vi "PH_Beckhoff_StepMot.Action Configure.vi"(0 "VI in":refnum<vi>, 5 "error in":errorcluster) -> (14 "VI out":refnum<vi>, 19 "error out":errorcluster)   [LabVIEW 2014, in "PH_Beckhoff_StepMot.lvlib"]
uses:
  PH_Beckhoff_StepMot.lvlib
  PH_Beckhoff/PH_Beckhoff.lvlib
  PH_Basics/PH_Stepmotor_BaseClass/PH_Stepmotor_BaseClass.lvlib
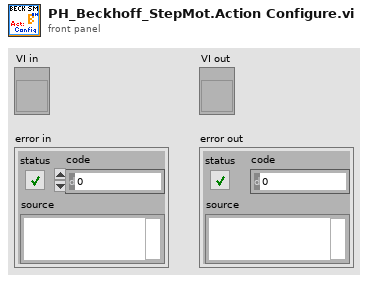
[diagram p1: front panel]
types:
  T1 = typedef "PH_Beckhoff.lvlib/PH_Beckhoff.i attribute.ctl" = cluster{"GUI Refs":T2, "operation?":bool, "Default Prdc Interval":i32, "Connection":T3, "AMS Net ID":T4, "Klemmencluster: # of":T5, "Values":T6, "IP":string, "Description":string, "configured?":bool, "Change Manager":cluster{"Detemination wanted?":bool, "Values changed at":cluster{"Sonderklemmen Inputs":i32[], "Analog Inputs":i32[], "Analog Outputs":i32[], "Digital Inputs":i32[], "Digital Outputs":i32[]}}, "Difference to handle an analog input as change":u32}
  T2 = typedef "PH_Beckhoff.lvlib/PH_Beckhoff.GUI Refs.ctl" = cluster{"ADS Error":refnum<vi>, "Values":refnum<vi>, "configured?":refnum<vi>, "Connection":refnum<vi>, "IP":refnum<vi>, "Prdc Int [ms]":refnum<vi>}
  T3 = typedef "PH_Beckhoff.lvlib/PH_Beckhoff.Connectivity.ctl" = cluster{"DLL?":bool, "Port?":bool, "Client?":bool, "Ping?":bool, "unsuccessful Pings":u32}
  T4 = typedef "Beckhoff - Driver np.lvlib/Beckhoff Access.ctl" = cluster{"DLL path":path, "AMS Net ID":cluster{"1st # of IP":u8, "2nd # of IP":u8, "3rd # of IP":u8, "4th # of IP":u8, "In Port":u8, "Out Port":u8}}
  T5 = typedef "Beckhoff - Driver np.lvlib/Klemmendeclarer.ctl" = cluster{"Offset due to Sonderklemms":u32, "analog Inputs":u32, "analog Outputs":u32, "digital Input Bits":u32, "digital Output Bits":u32}
  T6 = typedef "PH_Beckhoff.lvlib/PH_Beckhoff.Values.ctl" = cluster{"Sonderklemmen Inputs":T7, "Analog Inputs":T8, "Analog Outputs":T10, "Digital Inputs":T11, "Digital Outputs":T12}
  T7 = typedef "PH_Beckhoff.lvlib/PH_Beckhoff.Sonderklemmen Inputs.ctl" = cluster{"Total Length":u32, "Name":string, "Value":u64, "Quality":bool, "Service ID":i32, "Offset":u32, "Length":u32}[]
  T8 = typedef "PH_Beckhoff.lvlib/PH_Beckhoff.Analog Inputs.ctl" = cluster{"Name":string, "Value":u32, "Quality":bool, "Service ID":i32, "Sca Type":T9}[]
  T9 = typedef "PH_Beckhoff.lvlib/PH_Beckhoff.Scaling Type.ctl" = enum16{"none", "0 ... 15 Bit -> 0 ... 5", "0 ... 15 Bit -> 0 ... 10", "0 ... 15 Bit -> 0 ... 25", "0 ... 15 Bit -> 4 ... 20", "0 ... 15 Bit -> 0 ... 1", "0 ... 15 Bit -> 0 ... 20000", "0 ... 15 Bit -> 0 ... 24000"}
  T10 = typedef "PH_Beckhoff.lvlib/PH_Beckhoff.Analog Outputs.ctl" = cluster{"Name":string, "Value":u32, "Quality":bool, "Wanted Value":u32, "Service ID":i32, "Sca Type":T9}[]
  T11 = typedef "PH_Beckhoff.lvlib/PH_Beckhoff.Digital Inputs.ctl" = cluster{"Name":string, "Value":bool, "Quality":bool, "Service ID":i32, "inverted?":bool}[]
  T12 = typedef "PH_Beckhoff.lvlib/PH_Beckhoff.Digital Outputs.ctl" = cluster{"Name":string, "Value":bool, "Quality":bool, "Wanted Value":bool, "Service ID":i32, "inverted?":bool}[]
  T13 = typedef "PH_Beckhoff_StepMot.lvlib/PH_Beckhoff_StepMot.i attribute.ctl" = cluster{"Axes Settings":T14[], "GUI Refs":cluster{"Axes Settings":refnum<vi>, "Stati":refnum<vi>}, "Get Beckhoff Settings":bool}
  T14 = typedef "PH_Beckhoff_StepMot.lvlib/PH_Beckhoff_StepMot.Axis Cluster.ctl" = cluster{"Step Motor Configuration":T15, "To set?":bool, "Endswitch inverted?":bool}
  T15 = typedef "Beckhoff - Driver np.lvlib/Beckhoff.Step Motor - Motor Configuration.ctl" = cluster{"Feature Register":T16, "I max A [mA]":dbl, "I max B [mA]":dbl, "v min":u32, "v max":u32, "a max":u32, "I hold [%]":u32, "Steps/qp":u32, "Feature Register 2":T17}
  T16 = typedef "Beckhoff - Driver np.lvlib/Beckhoff.Step Motor - Feature Register 1.ctl" = cluster{"en Auto Start":bool, "en Auto Stop":bool, "dis Wd Timer":bool, "OP Mode 1":bool, "OP Mode 2":bool, "Ramp Type":bool, "inv Pos Feedback":bool, "en User Cur Table":bool, "en Latch Evt Clr Pos":bool, "en Multi Latch Vals":bool, "en Sign Disp*":bool, "Feedback Type*":bool, "en neg Gate Lock*":bool, "en pos Gate Lock*":bool, "dis Enc Fltr*":bool, "en Counter Mode*":bool}
  T17 = typedef "Beckhoff - Driver np.lvlib/Beckhoff.Step Motor - Feature Register 2.ctl" = cluster{"rev Homing Dir":bool, "en Decac Ramp":bool, "Latch Reg Pos":bool, "Show Idle":bool, "dis Ref Input 1":bool, "dis Ref Input 2":bool, "en ext Auto Start":bool, "N/A":bool, "N/A":bool, "N/A":bool, "N/A":bool, "N/A":bool, "en Clr Proc Data":bool, "en Man Ecl Tolerce*":bool, "rev Dig Input 1":bool, "rev Dig Input 2":bool}
  T18 = typedef "PH_Stepmotor_BaseClass.lvlib/PH_Stepmotor_BaseClass.i attribute.ctl" = cluster{"Device Error":errorcluster, "Axes PSDB Thread":cluster{"Ref":refnum<vi>, "Q-Ref":refnum<queue>, "Data Status":T19}, "Axes":T20[], "Axes PSDB Infos":cluster{"GUI Name":string, "PSDB Instance ID":i32, "PSDB Status Service ID":i32, "Axis":i32, "Class":string}[], "GUI Refs":T25}
  T19 = typedef "PH_PSDBWriter.lvlib/PH_PSDBWriter.Data Status.ctl" = i16
  T20 = typedef "PH_Stepmotor_BaseClass.lvlib/PH_Stepmotor_BaseClass.Axis Attributes.ctl" = cluster{"Settings":T21, "Endswitch?":bool, "DIM Service IDs":T23, "Activity":T24, "Configured?":bool, "Position":cluster{"Current":i32, "Target":i32}, "Position to set":cluster{"New?":bool, "Wanted":i32}, "Stop?":bool, "Reset?":bool, "Move?":bool, "Nothing connected?":bool}
  T21 = typedef "PH_Stepmotor_BaseClass.lvlib/PH_Stepmotor_BaseClass.Axis Settings.ctl" = cluster{"Sign change":bool, "Width":dbl, "Calibration":dbl, "Unit":string, "Motor Type":T22, "Unit Width":string, "Unit CF":string}
  T22 = typedef "PH_Stepmotor_BaseClass.lvlib/PH_Stepmotor_BaseClass.Motor Type.ctl" = enum16{"Unspecific", "OWIS 49.120.2633", "OWIS 49.060.1033", "OWIS 43.040.2558", "Diamond Motion 2200 series", "OWIS 49.120.266B.MV6", "Calorimeter", "Linear Stage 1", "MICOS VT-80", "MICOS VT-80 S", "Standa Rotstage nt0.95A", "PUF RA 320.200", "PUF RA 800.200", "PUF RA 800.400", "PUF RA 400.50", "1324.nn.800.50", "1324.n9c.800.50", "1324.nn.320.200", "1324.nn.400.200", "1324.nn.800.200", "1324.nn.400.50", "1324.8c9c.800.50", "1324.8c9c.400.200"}
  T23 = typedef "PH_Stepmotor_BaseClass.lvlib/PH_Stepmotor_BaseClass.Axis DIM Service IDs.ctl" = cluster{"Settings":i32, "Information":i32}
  T24 = typedef "PH_Stepmotor_BaseClass.lvlib/PH_Stepmotor_BaseClass.Axis Activity.ctl" = enum16{"No Information", "stopped", "running", "Failure", "Alarm", "stopped at backward ES", "stopped at foreward ES"}
  T25 = typedef "PH_Stepmotor_BaseClass.lvlib/PH_Stepmotor_BaseClass.GUI Refs.ctl" = cluster{"Axes Configuration":refnum<vi>, "Device Error":refnum<vi>, "Axes PSDB Infos":refnum<vi>}
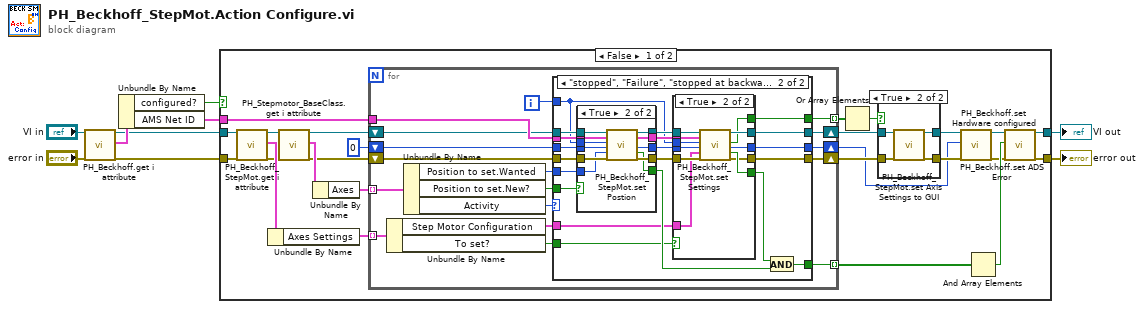
[diagram p0: block diagram]
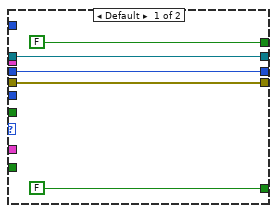
[diagram p3: hidden frame]
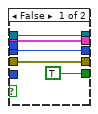
[diagram p4: hidden frame]
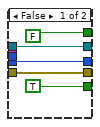
[diagram p5: hidden frame]
diagram:
  n1 = call "PH_Beckhoff.get i attribute.vi"("i ref in"="VI in", "error in (no error)"="error in") -> ("i ref out"=w4:refnum<vi>, "i attribute"=w7:T1, "error out"=w2:errorcluster)  [unwired: 15 in]
  n2 = Unbundle By Name(w7) -> ("configured?"=w1:bool, "AMS Net ID"=w6:T4)
  n3 = case shown="False" w1 {
    tunnel: [w31 w115] -> w9
    tunnel: [w30 w116] -> w8
    tunnel: w6 -> [w27 _]
    tunnel: w4 -> [w16 w116]
    tunnel: w2 -> [w13 w115]
    frame False {
      n4 = call "PH_Beckhoff_StepMot.get i attribute.vi"("i ref in"=w16, "error in (no error)"=w13) -> ("i ref out"=w15:refnum<vi>, "i attribute"=w32:T13, "error out"=w12:errorcluster)  [unwired: 15 in]
      n5 = Unbundle By Name(w32) -> ("Axes Settings"=w33:T14[])
      n6 = call "PH_Stepmotor_BaseClass.get i attribute.vi"("i ref in"=w15, "error in (no error)"=w12) -> ("i ref out"=w14:refnum<vi>, "i attribute"=w18:T18, "error out"=w11:errorcluster)  [unwired: 15 in]
      n7 = Unbundle By Name(w18) -> ("Axes"=w17:T20[])
      n8 = for {
        tunnel: w27 -> [w57]
        shift-right: [w53] -> w25
        shift-left: w11 -> [w56]
        shift-right: [w54] -> w10
        shift-left: 0 ("ADS Error out") -> [w55]
        tunnel: w33 -> [w43] mode=indexing
        shift-right: [w51] -> w22
        shift-left: w14 -> [w52]
        tunnel: [w44] -> w34 mode=indexing
        tunnel: [w50] -> w20 mode=indexing
        tunnel: w17 -> [w49] mode=indexing
        i -> [w46]
        n9 = Unbundle By Name(w43) -> ("Step Motor Configuration"=w42:T15, "To set?"=w41:bool)
        n10 = Unbundle By Name(w49) -> ("Position to set.Wanted"=w48:i32, "Position to set.New?"=w47:bool, "Activity"=w45:T24)
        n11 = case shown="\"stopped\", \"Failure\", \"stopped at backward ES\", \"stopped at foreward ES\"" w45 {
          tunnel: w57 -> [_ w78]
          tunnel: w56 -> [w61 w73]
          tunnel: w55 -> [w59 w77]
          tunnel: [w59 w82] -> w54
          tunnel: w42 -> [_ w64]
          tunnel: [w61 w81] -> w53
          tunnel: w52 -> [w62 w72]
          tunnel: [w62 w80] -> w51
          tunnel: [FALSE w66] -> w44
          tunnel: w46 -> [_ w68]
          tunnel: [FALSE ("Settings changed?") w79] -> w50
          tunnel: w48 -> [_ w76]
          tunnel: w47 -> [_ w69]
          tunnel: w41 -> [_ w63]
          frame Default {
          }
          frame "stopped", "Failure", "stopped at backward ES", "stopped at foreward ES" {
            n12 = case shown="True" w69 {
              tunnel: w78 -> [w85 w93]
              tunnel: w77 -> [w84 w92]
              tunnel: w68 -> [_ w94]
              tunnel: w76 -> [_ w91]
              tunnel: [w87 w97] -> w75
              tunnel: [w86 w95] -> w74
              tunnel: w73 -> [w86 w96]
              tunnel: w72 -> [w87 w98]
              tunnel: [w85 w90] -> w71
              tunnel: [w84 w89] -> w70
              tunnel: [TRUE ("ok?") w88] -> w67
              frame False {
              }
              frame True {
                n13 = call "PH_Beckhoff_StepMot.set Postion.vi"("VI in"=w98, "AMS Net ID"=w93, "Axis"=w94, "ADS Error in"=w92, "Wanted Position"=w91, "error in (no error)"=w96) -> ("VI out"=w97:refnum<vi>, "AMS Net ID out"=w90:T4, "ADS Error out"=w89:i32, "ok?"=w88:bool, "error out"=w95:errorcluster)  [unwired: 9 in]
              }
            }
            n14 = case shown="True" w63 {
              tunnel: w71 -> [_ w114]
              tunnel: w74 -> [w103 w113]
              tunnel: [TRUE w109] -> w65
              tunnel: w70 -> [w102 w112]
              tunnel: [w102 w111] -> w82
              tunnel: [w103 w108] -> w81
              tunnel: w64 -> [_ w110]
              tunnel: w75 -> [w100 w107]
              tunnel: [w100 w106] -> w80
              tunnel: w68 -> [_ w104]
              tunnel: [FALSE ("Settings changed?") w105] -> w79
              frame False {
              }
              frame True {
                n15 = call "PH_Beckhoff_StepMot.set Settings.vi"("VI in"=w107, "AMS Net ID in"=w114, "Axis"=w104, "ADS Error in"=w112, "Step Motor Configuration"=w110, "error in (no error)"=w113) -> ("VI out"=w106:refnum<vi>, "Settings changed?"=w105:bool, "ADS Error out"=w111:i32, "ok?"=w109:bool, "error out"=w108:errorcluster)  [unwired: 8 in, 1 out]
              }
            }
            n16 = And(x=w65, y=w67) -> (x .and. y?=w66:bool)
          }
        }
      }
      n17 = Or Array Elements(Boolean array=w20) -> (logical OR=w19:bool)
      n18 = case shown="True" w19 {
        tunnel: w25 -> [w35 w40]
        tunnel: [w35 w39] -> w23
        tunnel: w22 -> [w36 w38]
        tunnel: [w36 w37] -> w21
        frame False {
        }
        frame True {
          n19 = call "PH_Beckhoff_StepMot.set Axis Settings to GUI.vi"("VI in"=w38, "error in (no error)"=w40) -> ("VI out"=w37:refnum<vi>, "error out"=w39:errorcluster)  [unwired: 16 in]
        }
      }
      n20 = call "PH_Beckhoff.set ADS Error.vi"("i ref in"=w21, "ADS Error"=w10, "error in"=w23) -> ("i ref out"=w26:refnum<vi>, "error out"=w24:errorcluster)  [unwired: 15 in]
      n21 = And Array Elements(Boolean array=w34) -> (logical AND=w29:bool)
      n22 = call "PH_Beckhoff.set Hardware configured.vi"("i ref in"=w26, "Hardware configured?"=w29, "error in"=w24) -> ("i ref out"=w30:refnum<vi>, "error out"=w31:errorcluster)  [unwired: 15 in]
    }
    frame True {
    }
  }
  "error out" <- w9
  "VI out" <- w8
